vi "Join Numbers.vi"(11 "Array of 4 U8":u8[](array[numeric]) format="%02x") -> (3 "Single-Precision Float":sgl)   [LabVIEW 2011]
doc: "This VI computes IEEE 754-2008 from an array of 4 U8"
panel:
  out "Error Out":errorcluster
  in  "Error In":errorcluster
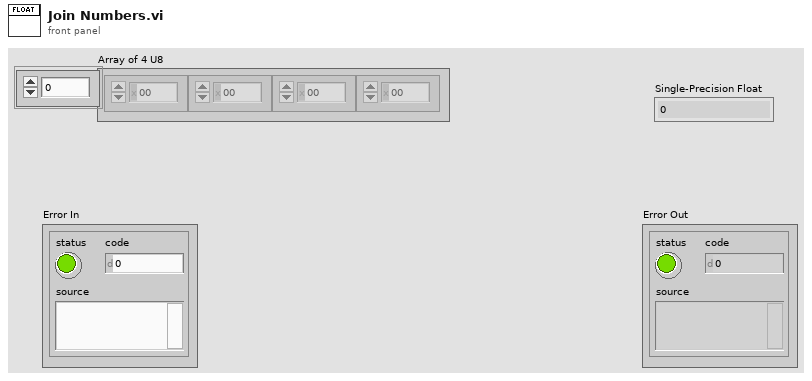
[diagram p1: front panel]
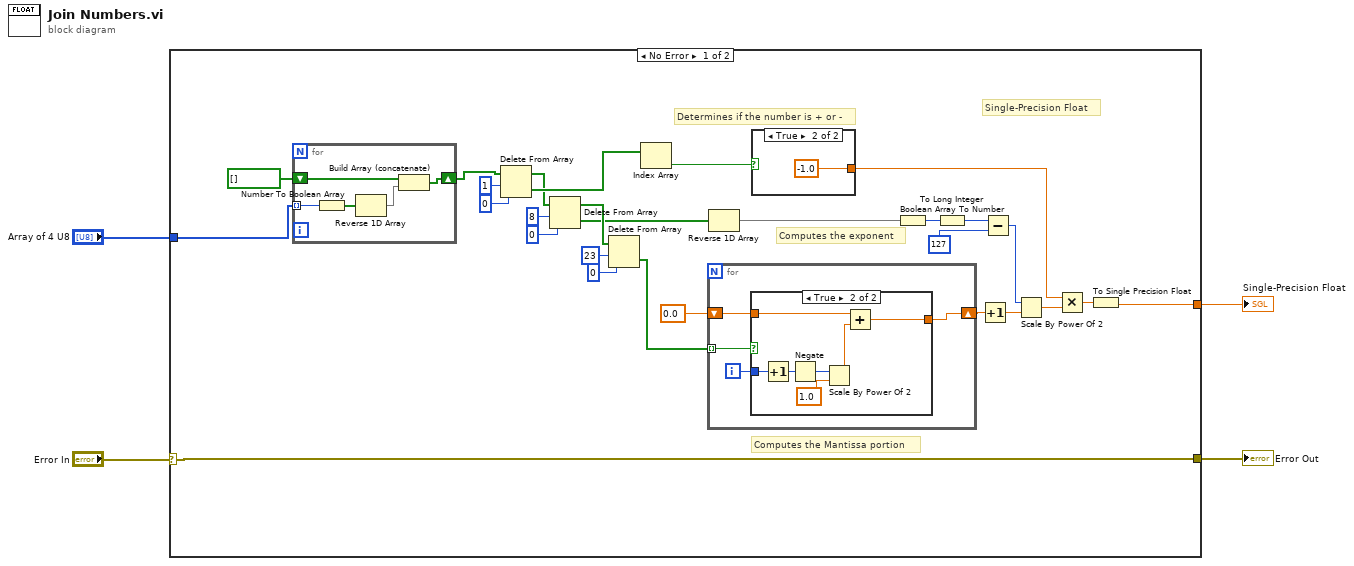
[diagram p0: block diagram]
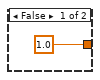
[diagram p2: hidden frame]
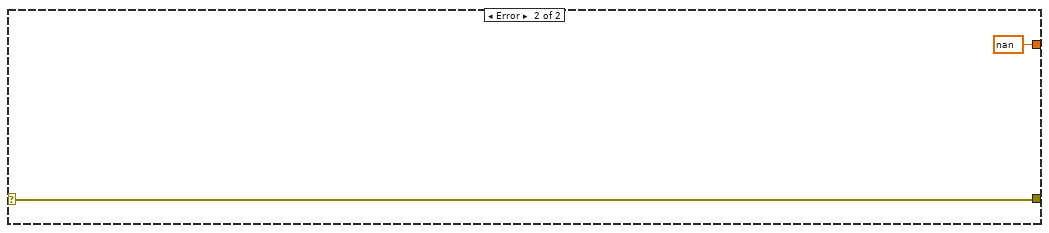
[diagram p4: hidden frame]
diagram:
  n1 = case shown="No Error" "Error In" {
    selector: "Error In" -> [w5 w53]
    tunnel: [w32 sgl nan] -> w4
    tunnel: "Array of 4 U8" -> [w31 _]
    tunnel: [w5 w53] -> w1
    frame No Error {
      # "Single-Precision Float"
      # "Computes the Mantissa portion"
      # "Computes the exponent"
      # "Determines if the number is + or -"
      n2 = for {
        tunnel: w31 -> [w51] mode=indexing
        shift-right: [w49] -> w30
        shift-left: bool[] [] -> [w50]
        n3 = Number To Boolean Array(number=w51) -> (Boolean array=w48:bool[])
        n4 = Reverse 1D Array(array=w48) -> (reversed array=w47:bool[])
        n5 = Build Array (concatenate)(w50, w47) -> (w49:bool[])
      }
      n6 = Delete From Array(array=w30, length=1, index=0) -> (deleted portion=w18:bool[], array with subset deleted=w16:bool[])
      n7 = Delete From Array(array=w16, length=8, index=0) -> (deleted portion=w8:bool[], array with subset deleted=w14:bool[])
      n8 = Delete From Array(array=w14, length=23, index=0) -> (deleted portion=w12:bool[])  [unwired: 1 out]
      n9 = Index Array(array=w18) -> (element=w17:bool)  [unwired: 1 in]
      n10 = for {
        shift-right: [w36] -> w28
        shift-left: 0.0 -> [w37]
        tunnel: w12 -> [w35] mode=indexing
        i -> [w38]
        n11 = case shown="True" w35 {
          tunnel: w38 -> [_ w46]
          tunnel: w37 -> [w39 w42]
          tunnel: [w39 w40] -> w36
          frame False {
          }
          frame True {
            n12 = Increment(x=w46) -> (x+1=w45:i32)
            n13 = Negate(x=w45) -> (-x=w44:i32)
            n14 = Scale By Power Of 2(n=w44, x=1.0) -> (x*2^n=w41:dbl)
            n15 = Add(x=w42, y=w41) -> (x+y=w40:dbl)
          }
        }
      }
      n16 = Reverse 1D Array(array=w8) -> (reversed array=w7:bool[])
      n17 = case shown="True" w17 {
        tunnel: [1.0 -1.0] -> w23
        frame False {
        }
        frame True {
        }
      }
      n18 = Boolean Array To Number(Boolean array=w7) -> (number=w21:u32)
      n19 = To Long Integer(number=w21) -> (32bit integer=w20:i32)
      n20 = Increment(x=w28) -> (x+1=w26:dbl)
      n21 = Subtract(x=w20, y=127) -> (x-y=w22:i32)
      n22 = Scale By Power Of 2(n=w22, x=w26) -> (x*2^n=w25:dbl)
      n23 = Multiply(x=w23, y=w25) -> (x*y=w24:dbl)
      n24 = To Single Precision Float(number=w24) -> (single precision float=w32:sgl)
    }
    frame Error {
    }
  }
  "Single-Precision Float" <- w4
  "Error Out" <- w1
